vi "ELVIS III v1.0 AI Read Bank A.vi"(8 "error in (no error)":errorcluster, 10 "AI.A.CNFG":u8[](array[numeric])=[0, 0, 0, 0, 0, 0, 0, 0, 0, 0, 0, 0], 11 "Refnum in":T1) -> (0 "error out":errorcluster)   [LabVIEW 2021]
uses:
  <vilib>/myRIO/Common/Instrument Driver Framework/ELVIS III v1.0/AI/typedefs/ELVIS III AI Channels FPGA Reference.ctl
  <vilib>/Utility/error.llb/Error Cluster From Error Code.vi
  <vilib>/rvi/errors/niLvFpgaAdjustHostInterfaceError.vi
  <vilib>/rvi/interface/nirviReadWriteControl/nirviReadWriteControl.xnode
  <vilib>/rvi/interface/Simulation/niFpgaSimulationCallBeginRW.vi
  NiFpgaLv.dll
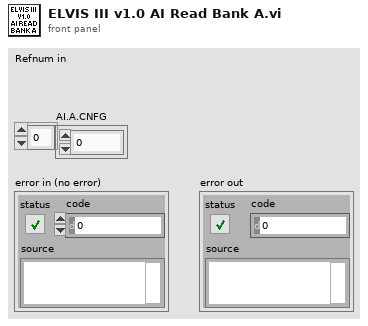
[diagram p1: front panel]
types:
  T1 = typedef "ELVIS III AI Channels FPGA Reference.ctl" = refnum<k20>
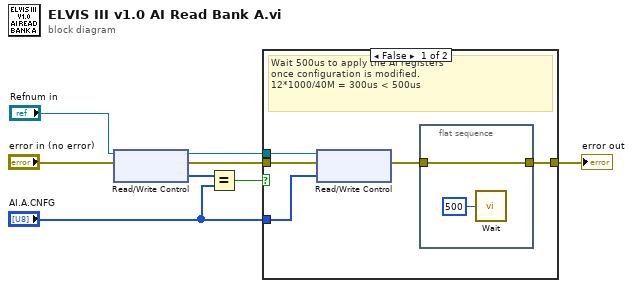
[diagram p0: block diagram]
diagram:
  n1 = xnode "Read/Write Control"("FPGA VI Reference In"="Refnum in", "error in"="error in (no error)") -> ("FPGA VI Reference Out"=w5:T1, "error out"=w4:errorcluster, "AI.A.CNFG"=w6:u8[])
  n2 = Equal?(x=w6, y="AI.A.CNFG") -> (x = y?=w3:bool)
  n3 = case shown="False" w3 {
    tunnel: w5 -> [w13 _]
    tunnel: w4 -> [w11 w16]
    tunnel: "AI.A.CNFG" -> [w12 _]
    tunnel: [w10 w16] -> w1
    frame False {
      # "Wait 500us to apply the AI registers \nonce configuration is modified.\n12*1000/40M = 300us < 500us"
      n4 = xnode "Read/Write Control"("FPGA VI Reference In"=w13, "error in"=w11, "AI.A.CNFG"=w12) -> ("error out"=w9:errorcluster)  [unwired: 1 out]
      n5 = flat-sequence {
        tunnel: [w15] -> w10
        tunnel: w9 -> [w15]
        frame #0 {
          n6 = call "Wait"("Count(uSec)"=u32 500) -> ()  [unwired: 1 out]
        }
      }
    }
    frame True {
    }
  }
  "error out" <- w1
